vi "Derivada_x_y.vi"(6 "Paso":dbl, 9 "Y":dbl[](array[numeric]), 10 "Tiempo":dbl, 11 "X":dbl[](array[numeric])) -> (2 "Yp":dbl[](array[numeric]), 3 "Xp":dbl[](array[numeric]))   [LabVIEW 2011]
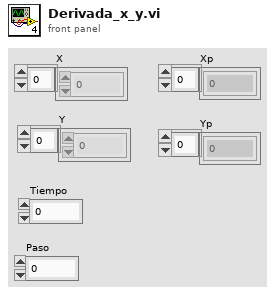
[diagram p1: front panel]
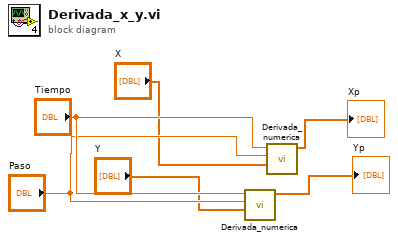
[diagram p0: block diagram]
diagram:
  n1 = call "Derivada_numerica.vi"("Funcion"="Y", "Paso"="Paso", "Tiempo"="Tiempo") -> ("Derivada"=→"Yp":dbl[])  [unwired: 8 in]
  n2 = call "Derivada_numerica.vi"("Funcion"="X", "Paso"="Paso", "Tiempo"="Tiempo") -> ("Derivada"=→"Xp":dbl[])  [unwired: 8 in]
